vi "SS_Calibration.vi"(9 "Raw value":sgl[](array[numeric])=[0.0, 0.0, 0.0, 0.0, 0.0, 0.0, 0.0, 0.0, 0.0, 0.0, 0.0, 0.0, 0.0, 0.0, 0.0, 0.0], 10 "Calibration value":sgl[](array[numeric])=[0.0, 0.0, 0.0, 0.0, 0.0, 0.0, 0.0, 0.0, 0.0, 0.0, 0.0, 0.0, 0.0, 0.0, 0.0, 0.0], 11 "Offset Value":sgl[](array[numeric])=[0.0, 0.0, 0.0, 0.0, 0.0, 0.0, 0.0, 0.0, 0.0, 0.0, 0.0, 0.0, 0.0, 0.0, 0.0, 0.0]) -> (2 "Calibrated data out":sgl[](array[numeric]) format="%.27g")   [LabVIEW 2016]
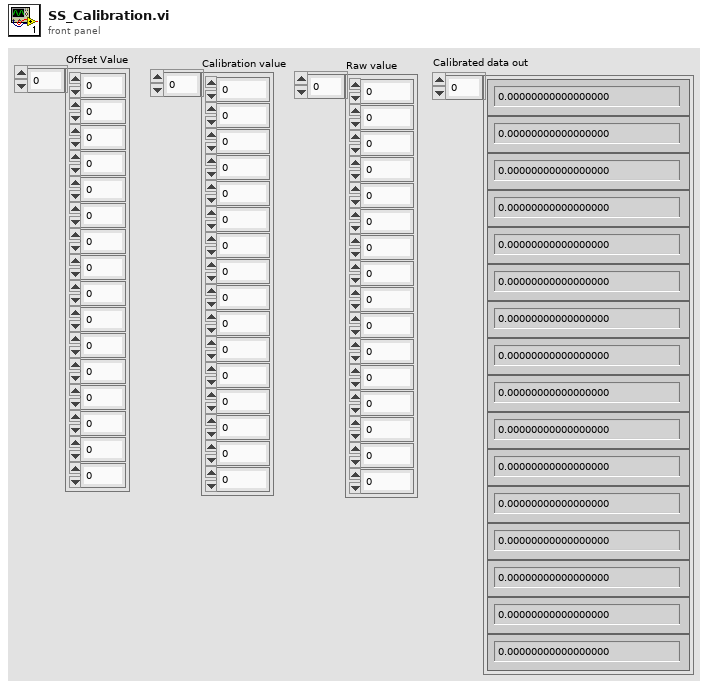
[diagram p1: front panel]
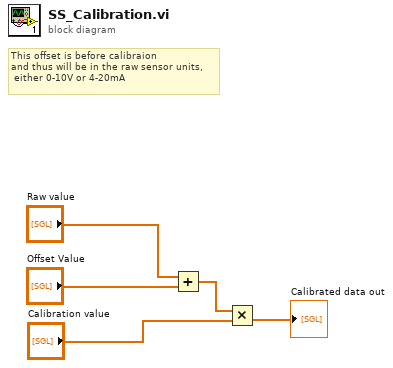
[diagram p0: block diagram]
diagram:
  # "This offset is before calibraion \nand thus will be in the raw sensor units,\n either 0-10V or 4-20mA"
  n1 = Add(x="Raw value", y="Offset Value") -> (x+y=w5:sgl[])
  n2 = Multiply(x=w5, y="Calibration value") -> (x*y=→"Calibrated data out":sgl[])
